vi "Read Attributes.vi"(11 "Abstract Message Msg":refnum<class "Abstract Message Msg.lvclass">) -> (2 "Payload":cluster{"Msg Data String":string})   [LabVIEW 2020, in "Nested Actor.lvlib" / "Abstract Message Msg.lvclass"]
uses:
  Abstract Message Msg.lvclass
  Abstract Message Msg.lvclass/Abstract Message Msg.ctl
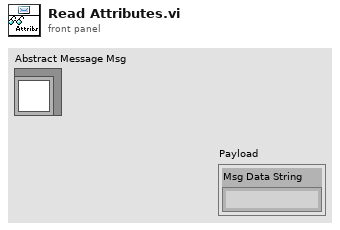
[diagram p1: front panel]
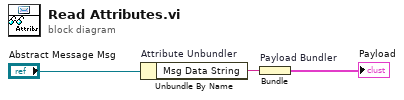
[diagram p0: block diagram]
diagram:
  n1 = Unbundle By Name "Attribute Unbundler"("Abstract Message Msg") -> ("Msg Data String"=w1:string)
  n2 = Bundle "Payload Bundler"("Msg Data String"=w1) -> (→"Payload":cluster{"Msg Data String":string})  [unwired: 1 in]
